vi "Init.vi"(8 "error in (no error)":errorcluster, 10 "Queries":refnum<class "CConfig Query.lvclass">[](array[class])) -> (0 "error out":errorcluster, 3 "Step In Query out":refnum<class "CConfig Query.lvclass">)   [LabVIEW 2013, in "Composite Query.lvclass"]
doc: "Copyright 2018, Carya Automatisering, Wiebe Walstra."
uses:
  Composite Query.lvclass
  CConfig Query.lvclass
  Composite Query.lvclass/Composite Query.ctl
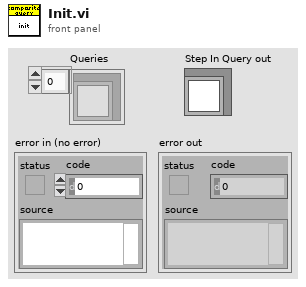
[diagram p1: front panel]
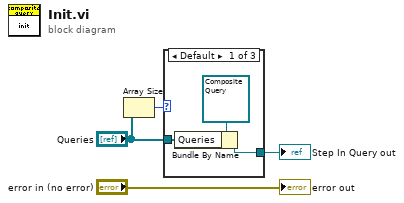
[diagram p0: block diagram]
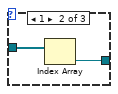
[diagram p2: hidden frame]
diagram:
  n1 = Array Size(array="Queries") -> (size(s)=w1:i32)
  n2 = case shown="Default" w1 {
    tunnel: [w6 w8 _] -> w3
    tunnel: "Queries" -> [w5 w9 _]
    frame Default {
      n3 = Bundle By Name(cluster=refnum<class "Composite Query.lvclass"> refnum ("Step In Query in"), "Queries"=w5) -> (w6:refnum<class "Composite Query.lvclass">)
    }
    frame 1 {
      n4 = Index Array(array=w9) -> (element=w8:refnum<class "CConfig Query.lvclass">)  [unwired: 1 in]
    }
    frame 0 {
    }
  }
  "Step In Query out" <- w3
  "error out" <- "error in (no error)"
